vi "Greenhouse Fuzzy Logic Control System.vi"() -> ()   [LabVIEW 2024]
uses:
  <vilib>/addons/Fuzzy Logic/FL Fuzzy Controller (MIMO).vi
  <vilib>/addons/Fuzzy Logic/NI_Fuzzy_Logic_API.lvlib
  <vilib>/httpClient/LabVIEWHTTPClient.lvlib
panel:
  in  "Light Intensity. (LUX)":dbl(slide) scale=0.0..3000.0
  out "Element":dbl
  in  "Value No.":i32
  out "Array":dbl[](array[numeric])
  out "array":dbl[][](array[numeric])
  out "URL":string
  in  "Num of Values":dbl
  in  "Field No.":dbl
  out "Body":string
  out "String":string
  out "Water Spills (%)":u8(slide) scale=0.0..100.0
  out "Electric Roof (%)":u8(slide) scale=0.0..100.0
  in  "Hum. (%)":dbl(slide) scale=0.0..100.0
  in  "Temp. (C)":dbl(slide) scale=0.0..80.0
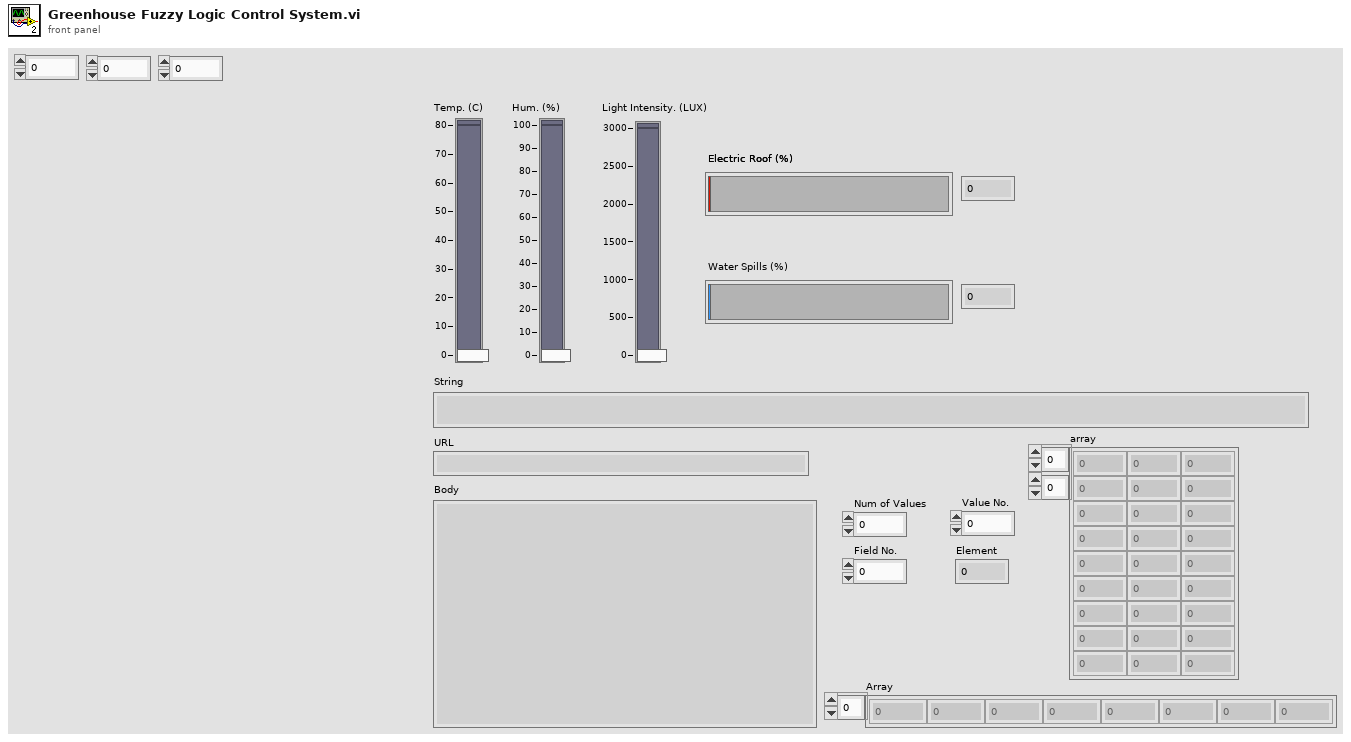
[diagram p1: front panel]
types:
  T1 = typedef "NI_Fuzzy_Logic_API.lvlib/FL System.ctl" = cluster{"input variables":T2[], "output variables":T2[], "rules":T5[], "defuzzification method":T11, "description":string, "user MF interpolating polynomials":T12[]}
  T2 = typedef "NI_Fuzzy_Logic_API.lvlib/FL Variable.ctl" = cluster{"name":string, "range":dbl[], "MFs":T3[]}
  T3 = typedef "NI_Fuzzy_Logic_API.lvlib/FL Membership Function.ctl" = cluster{"name":string, "shape":T4, "points":dbl[], "color":u32, "user-defined shape index":i32}
  T4 = typedef "NI_Fuzzy_Logic_API.lvlib/FL Membership Function Shape.ctl" = u16
  T5 = typedef "NI_Fuzzy_Logic_API.lvlib/FL Rule.ctl" = cluster{"antecedents":T6[], "antecedent connective":T8, "consequents":T9[], "consequent implication":T10, "degree of support":dbl}
  T6 = typedef "NI_Fuzzy_Logic_API.lvlib/FL Antecedent.ctl" = cluster{"Var Index":i32, "MF Index":i32, "Cond":T7}
  T7 = typedef "NI_Fuzzy_Logic_API.lvlib/FL Modifier.ctl" = u16
  T8 = typedef "NI_Fuzzy_Logic_API.lvlib/FL Antecedent Connective.ctl" = u16
  T9 = typedef "NI_Fuzzy_Logic_API.lvlib/FL Consequent.ctl" = cluster{"Var Index":i32, "MF Index":i32, "Cond":T7}
  T10 = typedef "NI_Fuzzy_Logic_API.lvlib/FL Consequent Implication.ctl" = u16
  T11 = typedef "NI_Fuzzy_Logic_API.lvlib/FL Defuzzification.ctl" = u16
  T12 = typedef "NI_Fuzzy_Logic_API.lvlib/FL Interpolating polynomials.ctl" = cluster{"X":dbl[], "Y":dbl[], "Y(x) coeff":dbl[][], "X(y) coeff":dbl[][], "Area(y) coeff":dbl[][], "coa_x(y) coeff":dbl[][]}
  T13 = typedef "LabVIEWHTTPClient.lvlib/ClientHandle.ctl" = refnum<k1>
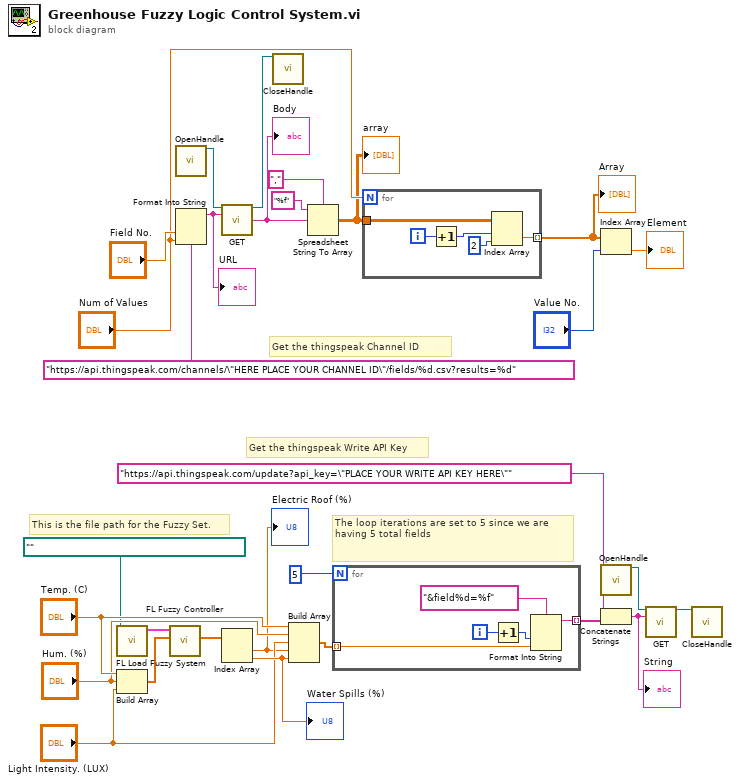
[diagram p0: block diagram]
diagram:
  # "Get the thingspeak Channel ID"
  # "Get the thingspeak Write API Key"
  # "The loop iterations are set to 5 since we are having 5 total fields"
  # "This is the file path for the Fuzzy Set."
  n1 = call <vilib>:"FL Load Fuzzy System.vi"("file path"=path "") -> ("fuzzy system out"=w29:T1)  [unwired: 9 in, 1 out]
  n2 = Build Array("Temp. (C)", "Hum. (%)", "Light Intensity. (LUX)") -> (w28:dbl[])
  n3 = call-poly <vilib>:"FL Fuzzy Controller.vi"("input values"=w28, "fuzzy system in"=w29) -> ("output values"=w27:dbl[])  [unwired: 5 in, 4 out]
  n4 = call <vilib>:"OpenHandle.vi"() -> ("client handle out"=w17:T13)  [unwired: 14 in, 1 out]
  n5 = Format Into String(format string="https://api.thingspeak.com/channels/\"HERE PLACE YOUR CHANNEL ID\"/fields/%d.csv?results=%d" ("url"), "Field No.", "Num of Values") -> (resulting string=w13:string)  [unwired: 2 in, 1 out]
  "URL" <- w13
  n6 = call <vilib>:"GET.vi"("client handle"=w17, "url"=w13) -> ("client handle out"=w16:T13, "body"=w12:string)  [unwired: 10 in, 2 out]
  "Body" <- w12
  n7 = Index Array(array=w27) -> (element #1=w1:dbl, element #2=w3:dbl)  [unwired: 2 in]
  "Electric Roof (%)" <- w1
  "Water Spills (%)" <- w3
  n8 = call <vilib>:"CloseHandle.vi"("client handle"=w16) -> ()  [unwired: 14 in, 1 out]
  n9 = Build Array("Temp. (C)", "Hum. (%)", "Light Intensity. (LUX)", w1, w3) -> (w20:dbl[])
  n10 = Spreadsheet String To Array(delimiter (Tab)=",", format string="%f", spreadsheet string=w12) -> (array=w8:dbl[][])  [unwired: 1 in]
  "array" <- w8
  n11 = for {
    N: 5 -> [_]
    tunnel: w20 -> [w32] mode=indexing
    tunnel: [w31] -> w18 mode=indexing
    i -> [w34]
    n12 = Increment(x=w34) -> (x+1=w33:i32)
    n13 = Format Into String(format string="&field%d=%f", w33, w32) -> (resulting string=w31:string)  [unwired: 2 in, 1 out]
  }
  n14 = for {
    N: "Num of Values" -> [_]
    tunnel: w8 -> [w37]
    tunnel: [w38] -> w7 mode=indexing
    i -> [w39]
    n15 = Increment(x=w39) -> (x+1=w35:i32)
    n16 = Index Array(array=w37, index (row)=w35, index (col)=2 ("index")) -> (element=w38:dbl)
  }
  "Array" <- w7
  n17 = Index Array(array=w7, index="Value No.") -> (element=→"Element":dbl)
  n18 = call <vilib>:"OpenHandle.vi"() -> ("client handle out"=w25:T13)  [unwired: 14 in, 1 out]
  n19 = Concatenate Strings("https://api.thingspeak.com/update?api_key=\"PLACE YOUR WRITE API KEY HERE\"" ("string"), w18) -> (w24:string)
  "String" <- w24
  n20 = call <vilib>:"GET.vi"("client handle"=w25, "url"=w24) -> ("client handle out"=w26:T13)  [unwired: 10 in, 3 out]
  n21 = call <vilib>:"CloseHandle.vi"("client handle"=w26) -> ()  [unwired: 14 in, 1 out]
